vi "Run and wait.vi"(8 "错误输入":errorcluster, 9 "Script":string, 10 "Script Name":string="TSB_Script", 11 "VISA资源名称":refnum<visa-resource-name>) -> (0 "错误输出":errorcluster, 3 "VISA资源名称输出":refnum<visa-resource-name>)   [LabVIEW 2020]
uses:
  Global variable.vi
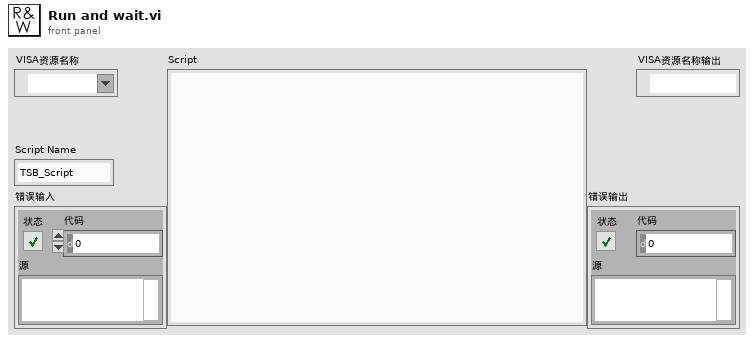
[diagram p1: front panel]
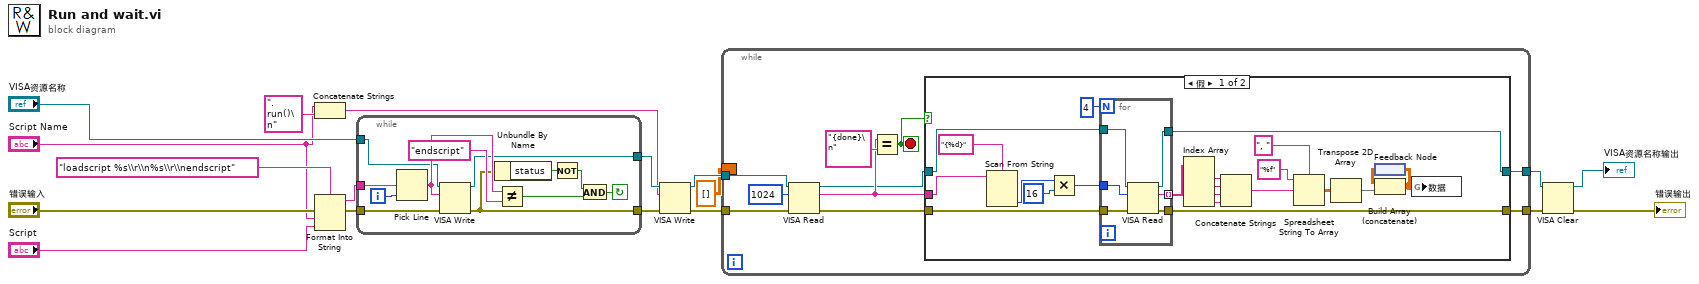
[diagram p0: block diagram]
diagram:
  n1 = Concatenate Strings("Script Name", ".run()\n" ("string")) -> (w8:string)
  n2 = Format Into String(format string="loadscript %s\\r\\n%s\\r\\nendscript", error in="错误输入", "Script Name", "Script") -> (resulting string=w16:string, error out=w13:errorcluster)  [unwired: 1 in]
  n3 = while {
    tunnel: w16 -> [w29]
    tunnel: "VISA资源名称" -> [w22]
    tunnel: w13 -> [w21]
    tunnel: [w20] -> w12
    tunnel: [w19] -> w11
    i -> [w30]
    stop <- w23 continue-if-true
    n4 = Pick Line(multi-line string=w29, line index=w30) -> (output string=w27:string)  [unwired: 1 in]
    n5 = VISA Write(VISA resource name=w22, write buffer=w27, error in (no error)=w21) -> (VISA resource name out=w19:refnum<visa-resource-name>, error out=w20:errorcluster)  [unwired: 1 out]
    n6 = Unbundle By Name(w20) -> ("status"=w26:bool)
    n7 = Not Equal?(x=w27, y="endscript") -> (x != y?=w24:bool)
    n8 = Not(x=w26) -> (.not. x?=w25:bool)
    n9 = And(x=w25, y=w24) -> (x .and. y?=w23:bool)
  }
  n10 = VISA Write(VISA resource name=w11, write buffer=w8, error in (no error)=w12) -> (VISA resource name out=w5:refnum<visa-resource-name>, error out=w4:errorcluster)  [unwired: 1 out]
  n11 = while {
    tunnel: w5 -> [w39]
    tunnel: w4 -> [w38]
    tunnel: [w34] -> w2
    tunnel: [w33] -> w3
    border: dbl[][] [] -> [_]
    stop <- w31 stop-if-true
    n12 = VISA Read(VISA resource name=w39, byte count=u32 1024 ("字节总数"), error in (no error)=w38) -> (VISA resource name out=w32:refnum<visa-resource-name>, read buffer=w36:string, error out=w35:errorcluster)  [unwired: 1 out]
    n13 = Equal?(x=w36, y="{done}\n") -> (x = y?=w31:bool)
    n14 = case shown="假" w31 {
      tunnel: w36 -> [w62 _]
      tunnel: w35 -> [w60 w69]
      tunnel: [w59 w69] -> w34
      tunnel: [w58 w70] -> w33
      tunnel: w32 -> [w57 w70]
      frame False {
        n15 = Scan From String(format string="{%d}" ("格式字符串"), input string=w62) -> (output 1=w55:i32)  [unwired: 3 in, 3 out]
        n16 = Multiply(x=w55, y=16) -> (x*y=w53:i32)
        n17 = for {
          N: 4 -> [_]
          tunnel: w60 -> [w68]
          tunnel: [w67] -> w59
          tunnel: [w66] -> w58
          tunnel: w57 -> [w65]
          tunnel: w53 -> [w64]
          tunnel: [w63] -> w47 mode=indexing
          n18 = VISA Read(VISA resource name=w65, byte count=w64, error in (no error)=w68) -> (VISA resource name out=w66:refnum<visa-resource-name>, read buffer=w63:string, error out=w67:errorcluster)  [unwired: 1 out]
        }
        n19 = Index Array(array=w47) -> (element #1=w46:string, element #2=w45:string, element #3=w44:string, element #4=w41:string)  [unwired: 4 in]
        n20 = Concatenate Strings(w46, w45, w44, w41) -> (w52:string)
        n21 = Spreadsheet String To Array(delimiter (Tab)=", " ("分隔符(Tab)"), format string="%f" ("格式字符串"), spreadsheet string=w52) -> (array=w49:dbl[][])  [unwired: 1 in]
        n22 = Transpose 2D Array(2D array=w49) -> (transposed array=w48:dbl[][])
        n23 = feedback #1() -> (w43:dbl[][])
        n24 = Build Array (concatenate)(w43, w48) -> (w42:dbl[][])
        n25 = feedback-in #1(w42) -> ()
        n26 = global write "Global variable.vi" "数据"(w42) -> ()
      }
      frame True {
      }
    }
  }
  n27 = VISA Clear(VISA resource name=w3, error in (no error)=w2) -> (VISA resource name out=→"VISA资源名称输出":refnum<visa-resource-name>, error out=→"错误输出":errorcluster)
